vi "Delete all buttons.vi"(0 "Display State In":T1={"Buttons Displayed"=0, "Button States"=[], "Button Size"=0, "Button Style"=enum."Classic", "Active Button"=0, "Force Regen?"=FALSE, "Tip String Ref"=refnum}, 9 "Container State":T3, 11 "error in (no error)":errorcluster) -> (4 "Display State Out":T1={"Buttons Displayed"=0, "Button States"=[], "Button Size"=0, "Button Style"=enum."Classic", "Active Button"=0, "Force Regen?"=FALSE, "Tip String Ref"=refnum}, 15 "error out":errorcluster)   [LabVIEW 2012, in "Toolbar.xctl"]
doc: "Clear the toolbar completely"
uses:
  Toolbar.xctl
  <vilib>/_xctls/Container State.ctl
  Toolbar State.ctl
  Button_Class/Button.lvclass
  Button_Class/Type Defs/Button Style.ctl
  <vilib>/_xctls/XControlSupport.lvlib
panel:
  # "Add Controls & Indicators that form the parameters of the method here. Hook them to the connector pane. Do not delete the controls & indicators that are already hooked to the connector pane.\n \nTo setup the parameters  for this method, right click on this item in the Project Tree & select \"Configure Method...\"."
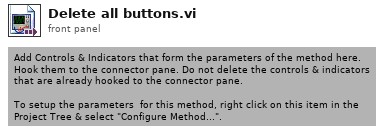
[diagram p1: front panel]
types:
  T1 = typedef "Toolbar.xctl/Toolbar State.ctl" = cluster{"Buttons Displayed":i32, "Button States":refnum<class "Button.lvclass">[], "Button Size":i32, "Button Style":T2, "Active Button":i32, "Force Regen?":bool, "Tip String Ref":refnum<vi>}
  T2 = typedef "Button.lvclass/Button Style.ctl" = enum16{"System", "Modern", "Classic", "Rounded", "Silver", "Ni Theme", "Metallic"}
  T3 = typedef "XControlSupport.lvlib/Container State.ctl" = cluster{"Indicator?":bool, "Run Mode?":bool, " Refnum":refnum<vi>}
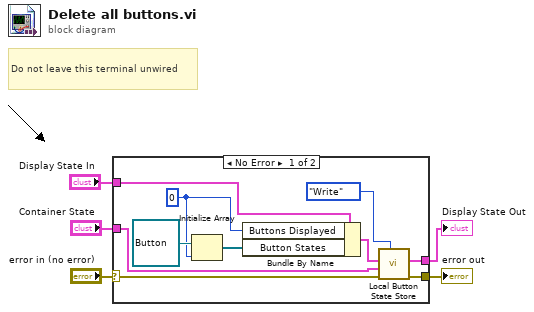
[diagram p0: block diagram]
diagram:
  # "Do not leave this terminal unwired"
  n1 = case shown="No Error" "error in (no error)" {
    selector: "error in (no error)" -> [w8 w17]
    tunnel: [w7 w17] -> w4
    tunnel: "Display State In" -> [w15 w16]
    tunnel: [w9 w16] -> w2
    tunnel: "Container State" -> [w6 _]
    frame No Error {
      w13 = 0 ("Buttons Displayed")
      n2 = Initialize Array(refnum<class "Button.lvclass"> refnum ("Button.lvclass"), w13) -> (w12:refnum<class "Button.lvclass">[])
      n3 = Bundle By Name(cluster=w15, "Buttons Displayed"=w13, "Button States"=w12) -> (w10:T1)
      n4 = call "Local Button State Store.vi"("Operation"=enum16{"Read", "Write"}."Write", "error in (no error)"=w8, "Container State"=w6, "Display State In"=w10) -> ("error out"=w7:errorcluster, "Display State Out"=w9:T1)  [unwired: 1 in, 5 out]
    }
    frame Error {
    }
  }
  "Display State Out" <- w2
  "error out" <- w4
